vi "Disable_Controls_during_Scan.vi"(8 "Error In":errorcluster, 9 "Control Reference Cluster Input":T1, 11 "Control State In":T2(ring)=enum."Disabled and Grayed Out") -> (0 "error out":errorcluster, 1 "Control Reference Cluster Output":T1)   [LabVIEW 2016]
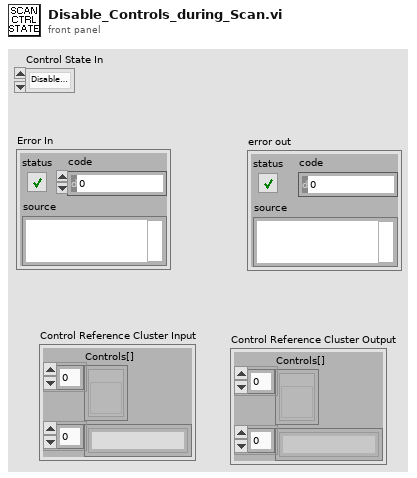
[diagram p1: front panel]
types:
  T1 = cluster{"Controls[]":refnum<vi>[], "Control Names":string[]}
  T2 = enum8{"Enabled", "Disabled", "Disabled and Grayed Out"}
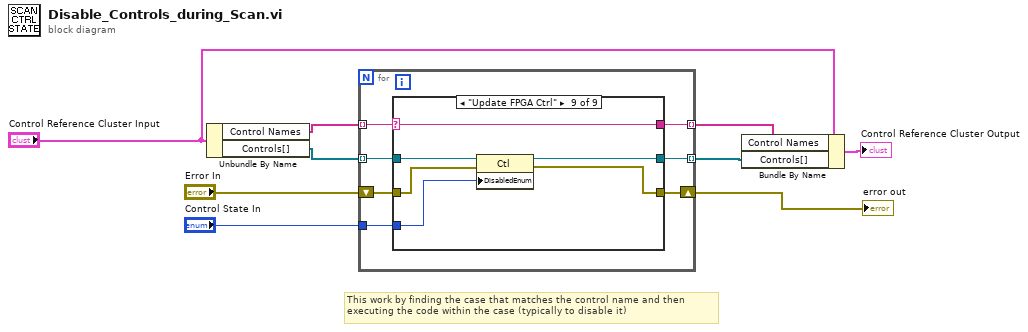
[diagram p0: block diagram]
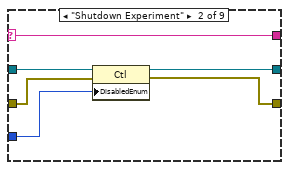
[diagram p3: hidden frame]
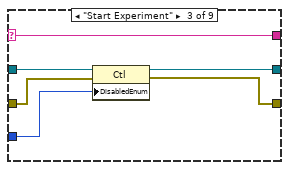
[diagram p4: hidden frame]
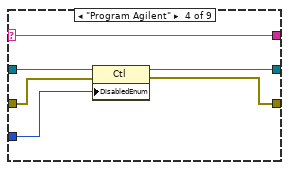
[diagram p5: hidden frame]
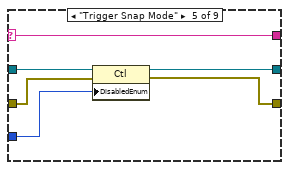
[diagram p6: hidden frame]
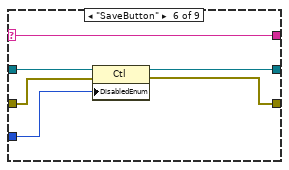
[diagram p7: hidden frame]
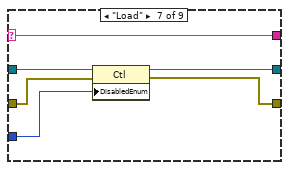
[diagram p8: hidden frame]
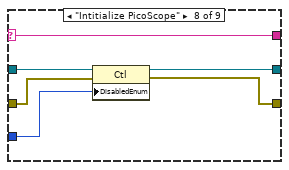
[diagram p9: hidden frame]
diagram:
  # "This work by finding the case that matches the control name and then\nexecuting the code within the case (typically to disable it)"
  n1 = Unbundle By Name("Control Reference Cluster Input") -> ("Control Names"=w6:string[], "Controls[]"=w5:refnum<vi>[])
  n2 = for {
    tunnel: w6 -> [w16] mode=indexing
    tunnel: "Control State In" -> [w14]
    tunnel: [w13] -> w4 mode=indexing
    shift-right: [w10] -> w7
    shift-left: "Error In" -> [w11]
    tunnel: w5 -> [w15] mode=indexing
    tunnel: [w12] -> w3 mode=indexing
    n3 = case shown="\"Update FPGA Ctrl\"" w16 {
      selector: w16 -> [w19 w24 w30 w36 w42 w48 w54 w60 w66]
      tunnel: w15 -> [w18 w21 w27 w33 w39 w45 w51 w57 w63]
      tunnel: w14 -> [_ w25 w31 w37 w43 w49 w55 w61 w67]
      tunnel: [w19 w24 w30 w36 w42 w48 w54 w60 w66] -> w13
      tunnel: [w18 w20 w26 w32 w38 w44 w50 w56 w62] -> w12
      tunnel: w11 -> [w17 w23 w29 w35 w41 w47 w53 w59 w65]
      tunnel: [w17 w22 w28 w34 w40 w46 w52 w58 w64] -> w10
      frame "False", Default {
      }
      frame "Shutdown Experiment" {
        n4 = property class="Ctl"(reference=w21, error in=w23, "DisabledEnum"=w25) -> (reference out=w20:refnum<vi>, error out=w22:errorcluster)
      }
      frame "Start Experiment" {
        n5 = property class="Ctl"(reference=w27, error in=w29, "DisabledEnum"=w31) -> (reference out=w26:refnum<vi>, error out=w28:errorcluster)
      }
      frame "Program Agilent" {
        n6 = property class="Ctl"(reference=w33, error in=w35, "DisabledEnum"=w37) -> (reference out=w32:refnum<vi>, error out=w34:errorcluster)
      }
      frame "Trigger Snap Mode" {
        n7 = property class="Ctl"(reference=w39, error in=w41, "DisabledEnum"=w43) -> (reference out=w38:refnum<vi>, error out=w40:errorcluster)
      }
      frame "SaveButton" {
        n8 = property class="Ctl"(reference=w45, error in=w47, "DisabledEnum"=w49) -> (reference out=w44:refnum<vi>, error out=w46:errorcluster)
      }
      frame "Load" {
        n9 = property class="Ctl"(reference=w51, error in=w53, "DisabledEnum"=w55) -> (reference out=w50:refnum<vi>, error out=w52:errorcluster)
      }
      frame "Intitialize PicoScope" {
        n10 = property class="Ctl"(reference=w57, error in=w59, "DisabledEnum"=w61) -> (reference out=w56:refnum<vi>, error out=w58:errorcluster)
      }
      frame "Update FPGA Ctrl" {
        n11 = property class="Ctl"(reference=w63, error in=w65, "DisabledEnum"=w67) -> (reference out=w62:refnum<vi>, error out=w64:errorcluster)
      }
    }
  }
  "error out" <- w7
  n12 = Bundle By Name(cluster="Control Reference Cluster Input", "Control Names"=w4, "Controls[]"=w3) -> (→"Control Reference Cluster Output":T1)
